vi "LoadData.vi"(5 "data files":path[](array[path]), 6 "error in (no error)":errorcluster, 7 "data type":T1, 8 "max amplitude of\noutput":dbl, 9 "CAR?":bool) -> (0 "error out":errorcluster, 1 "fs":dbl, 2 "# samples":i32, 3 "data":dbl[][](array[numeric]))   [LabVIEW 2017]
uses:
  DataType.ctl
panel:
  out "# series":i32
  # "Loads data from one or more *.continuous files or *.mat files (with format similar to the files in sEEG_Hippocampus, i.e. with fields 'data' and 'srate').\nSee the MATLAB script node for details on how the file(s) are loaded. \n\nOutput is a nChans x nSamples matrix. Files are concatentated along the channel dimension if multiple are provided (and must have the same number of samples).\n\nCan be extended by adding more types to DataType.ctl and providing methods to load them in the MATLAB script node."
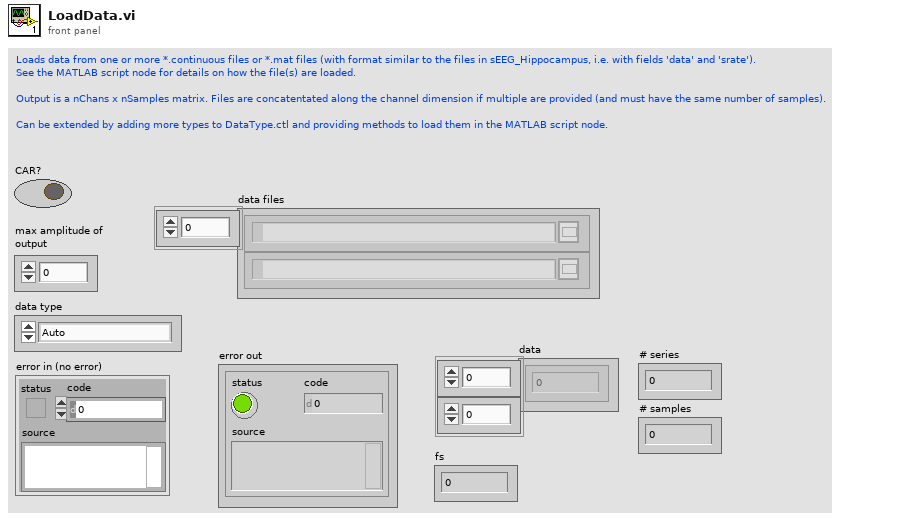
[diagram p1: front panel]
types:
  T1 = typedef "DataType.ctl" = enum16{"Auto", "Open Ephys", "Matlab (data and srate)"}
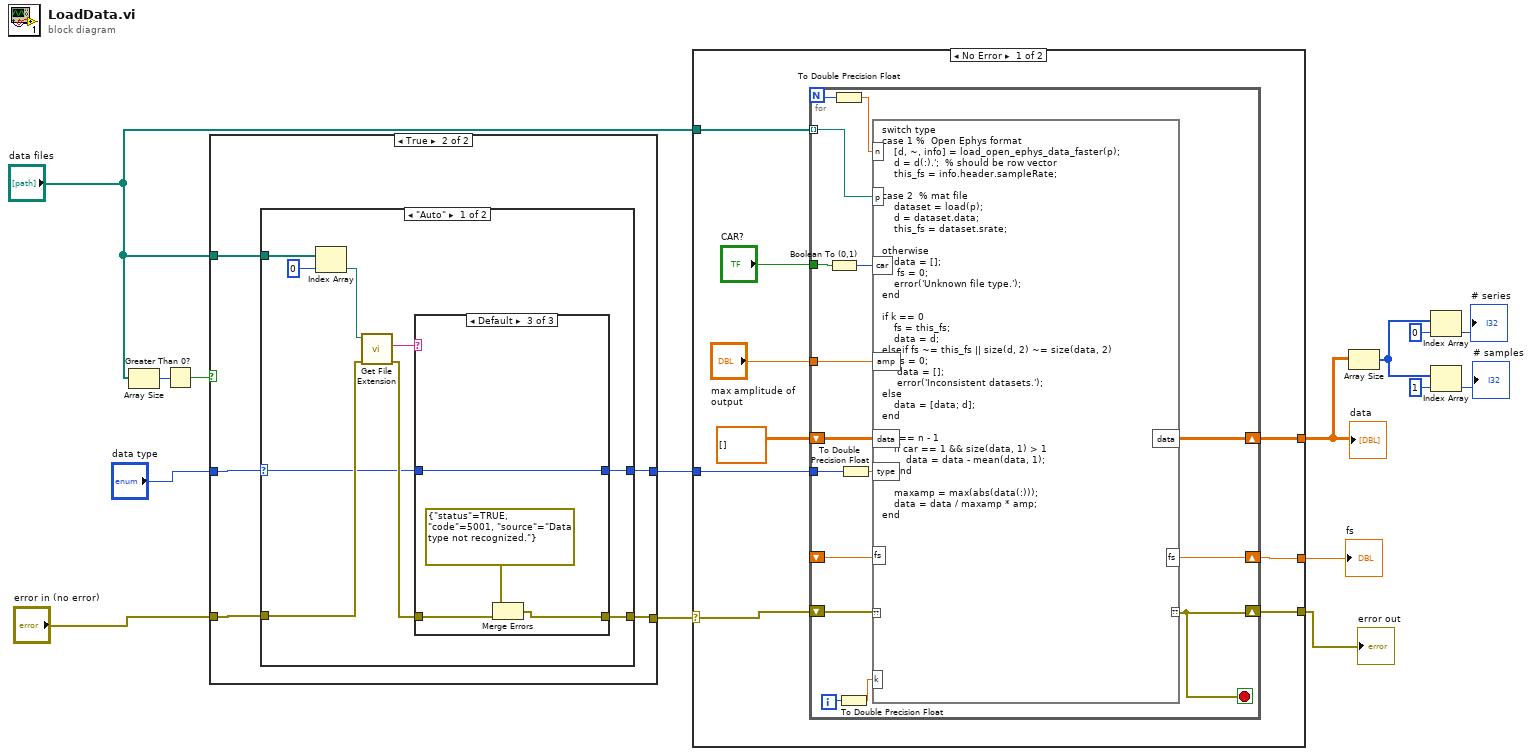
[diagram p0: block diagram]
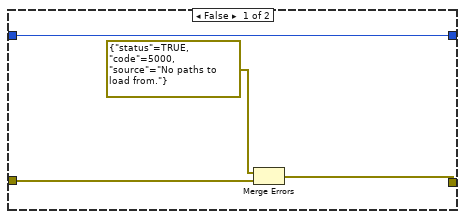
[diagram p2: hidden frame]
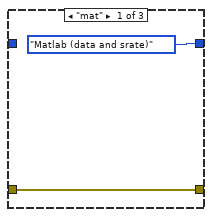
[diagram p3: hidden frame]
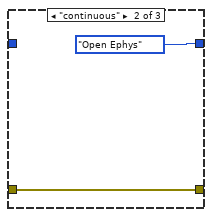
[diagram p4: hidden frame]
diagram:
  n1 = Array Size(array="data files") -> (size(s)=w14:i32)
  n2 = Greater Than 0?(x=w14) -> (x > 0?=w10:bool)
  n3 = case shown="True" w10 {
    tunnel: [w16 w24] -> w11
    tunnel: "data files" -> [_ w23]
    tunnel: "data type" -> [w16 w22]
    tunnel: "error in (no error)" -> [w19 w21]
    tunnel: [w18 w20] -> w9
    frame False {
      n4 = Merge Errors(errorcluster {"status"=TRUE, "code"=5000, "source"="No paths to load from."} ("error in (no error)"), w19) -> (w18:errorcluster)
    }
    frame True {
      n5 = case shown="\"Auto\"" w22 {
        selector: w22 -> [w25 w43]
        tunnel: [w27 w43] -> w24
        tunnel: w23 -> [w33 _]
        tunnel: w21 -> [w30 w42]
        tunnel: [w26 w42] -> w20
        frame "Auto" {
          n6 = Index Array(array=w33, index=0) -> (element=w31:path)
          n7 = call <vilib>:"Get File Extension.vi"("error in (no error)"=w30, "file"=w31) -> ("error out"=w28:errorcluster, "lowercase file extension"=w29:string)  [unwired: 5 in, 3 out]
          n8 = case shown="Default" w29 {
            tunnel: w28 -> [w34 w36 w41]
            tunnel: [DataType."Matlab (data and srate)" ("Enum") DataType."Open Ephys" ("Enum") w38] -> w27
            tunnel: [w34 w36 w40] -> w26
            tunnel: w25 -> [_ _ w38]
            frame "mat" {
            }
            frame "continuous" {
            }
            frame Default {
              n9 = Merge Errors(errorcluster {"status"=TRUE, "code"=5001, "source"="Data type not recognized."} ("error in"), w41) -> (w40:errorcluster)
            }
          }
        }
        frame "Matlab (data and srate)", Default {
        }
      }
    }
  }
  n10 = case shown="No Error" w9 {
    selector: w9 -> [w49 w69]
    tunnel: w11 -> [w52 _]
    tunnel: "data files" -> [w51 _]
    tunnel: [w50 w69] -> w7
    tunnel: [w48 _] -> w6
    tunnel: [w44 _] -> w8
    frame No Error {
      n11 = for {
        N -> [w54]
        tunnel: w51 -> [w68] mode=indexing
        tunnel: w52 -> [w67]
        shift-right: [w65] -> w50
        shift-left: w49 -> [w64]
        shift-right: [w62] -> w44
        shift-left: _ -> [w61]
        tunnel: "CAR?" -> [w58]
        tunnel: "max amplitude of\noutput" -> [w56]
        shift-right: [w60] -> w48
        shift-left: dbl[][] [] -> [w55]
        i -> [w59]
        stop <- w65 stop-if-true
        n12 = Boolean To (0,1)(Boolean=w58) -> (0, 1=w57:i16)
        n13 = To Double Precision Float(number=w54) -> (double precision float=w53:dbl)
        n14 = To Double Precision Float(number=w59) -> (double precision float=w63:dbl)
        n15 = To Double Precision Float(number=w67) -> (double precision float=w66:dbl)
        n16 = script code="switch type\ncase 1 %  Open Ephys format\n    [d, ~, info] = load_open_ephys_data_faster(p);\n    d = d(:).';  % should be row vector\n    this_fs = info.header.sampleRate;\n\ncase 2  % mat file\n    dataset = load(p);\n    d = dataset.data;\n    this_fs = dataset.srate;\n\notherwise\n    data = [];\n     fs = 0;\n    error('Unknown file type.');\nend\n\nif k == 0\n    fs = this_fs;\n    data = d;\nelseif fs ~= this_fs || size(d, 2) ~= size(data, 2)\n     fs = 0;\n     data = [];\n     error('Inconsistent datasets.');\nelse\n    data = [data; d]; \nend\n\nif k == n - 1\n    if car == 1 && size(data, 1) > 1\n        data = data - mean(data, 1);\n    end\n\n    maxamp = max(abs(data(:)));\n    data = data / maxamp * amp;\nend"("??"=w64, "p"=w68, "type"=w66, "k"=w63, "fs"=w61, "car"=w57, "amp"=w56, "data"=w55, "n"=w53) -> ("??"=w65:errorcluster, "data"=w60:dbl[][], "fs"=w62:dbl)
      }
    }
    frame Error {
    }
  }
  "data" <- w6
  "fs" <- w8
  "error out" <- w7
  n17 = Array Size(array=w6) -> (size(s)=w3:i32[])
  n18 = Index Array(array=w3, index=0) -> (element=→"# series":i32)
  n19 = Index Array(array=w3, index=1) -> (element=→"# samples":i32)
